vi "Configure Spectrum Emission Mask (Measurement Setup).vi"(0 "VISA resource name":refnum<visa-resource-name>, 5 "SEM Type (0:Integral Power)":i32(ring) items=["Integral Power", "Peak Power", "Fixed"], 7 "SEM Side (1:Upper Offset)":i32(ring)=1 items=["Upper and Lower", "Upper Offset", "Lower Offset"], 11 "error in (no error)":errorcluster) -> (4 "VISA resource name out":refnum<visa-resource-name>, 15 "error out":errorcluster)   [LabVIEW 2020, in "Anritsu Signal Analyzer Series.lvlib"]
doc: "Configures the SEM measurement parameters."
uses:
  Anritsu Signal Analyzer Series.lvlib
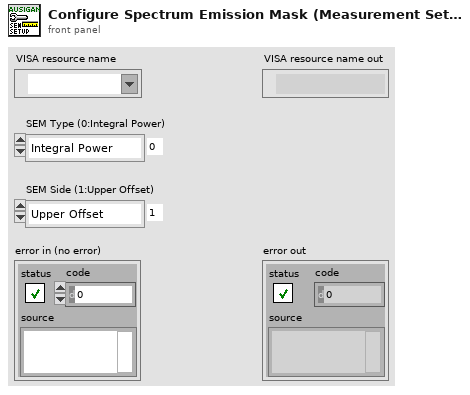
[diagram p1: front panel]
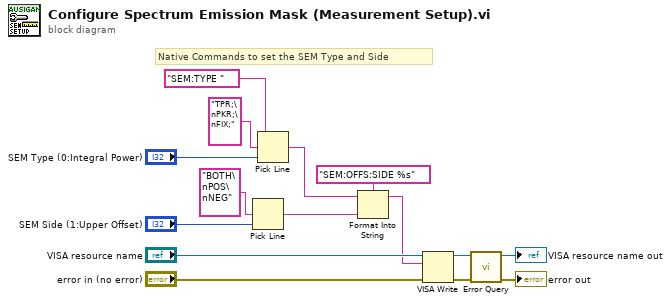
[diagram p0: block diagram]
diagram:
  # "Native Commands to set the SEM Type and Side"
  n1 = Pick Line(multi-line string="BOTH\nPOS\nNEG" ("複数行文字列"), line index="SEM Side (1:Upper Offset)") -> (output string=w1:string)  [unwired: 1 in]
  n2 = Pick Line(string ("")="SEM:TYPE " ("_CommandSet"), multi-line string="TPR;\nPKR;\nFIX;" ("複数行文字列"), line index="SEM Type (0:Integral Power)") -> (output string=w4:string)
  n3 = Format Into String(format string="SEM:OFFS:SIDE %s" ("_CommandSet"), initial string=w4, w1) -> (resulting string=w6:string)  [unwired: 1 in, 1 out]
  n4 = VISA Write(VISA resource name="VISA resource name", write buffer=w6, error in (no error)="error in (no error)") -> (VISA resource name out=w8:refnum<visa-resource-name>, error out=w7:errorcluster)  [unwired: 1 out]
  n5 = call "Error Query.vi"("error in (no error)"=w7, "VISA resource name"=w8) -> ("error out"=→"error out":errorcluster, "VISA resource name out"=→"VISA resource name out":refnum<visa-resource-name>)  [unwired: 6 in, 2 out]
